vi "PicoScope_Ini.vi"() -> ()   [LabVIEW 2018]
panel:
  out "Max Adc value":i16
  out "error out":errorcluster
  out "handle":i16
  out "Device Info":T1
  out "PicoScope Type":string
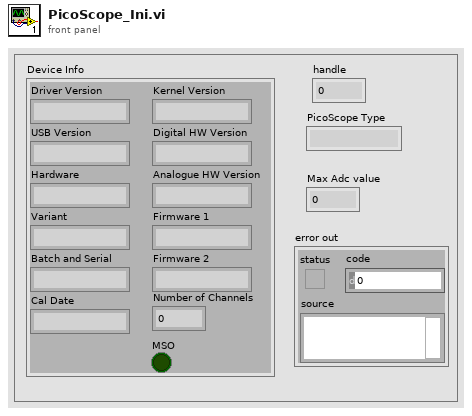
[diagram p1: front panel]
types:
  T1 = cluster{"Driver Version":string, "USB Version":string, "Hardware":string, "Variant":string, "Batch and Serial":string, "Cal Date":string, "Kernel Version":string, "Digital HW Version":string, "Analogue HW Version":string, "Firmware 1":string, "Firmware 2":string, "MSO":bool, "Number of Channels":i16}
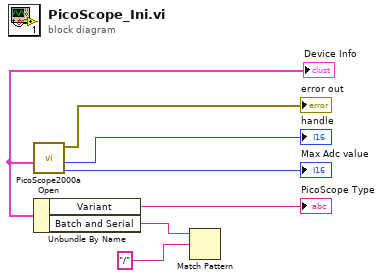
[diagram p0: block diagram]
diagram:
  n1 = call "PicoScope2000aOpen.vi"() -> ("Max Adc value"=→"Max Adc value":i16, "handle"=→"handle":i16, "error out"=→"error out":errorcluster, "Device Info"=w4:T1)  [unwired: 4 in]
  "Device Info" <- w4
  n2 = Unbundle By Name(w4) -> ("Variant"=→"PicoScope Type":string, "Batch and Serial"=w6:string)
  n3 = Match Pattern(string=w6, regular expression="/") -> ()  [unwired: 1 in, 4 out]
